vi "Filter Data.vi"(7 "k (0.7)":dbl=0.7 format="%#_13g", 10 "High Filter k (0.5)":dbl=0.5 format="%#_13g", 11 "Raw Acq Data in in":T1) -> (3 "Raw Acq Data out":T1)   [LabVIEW 2018, in "RT - Analysis.lvlib"]
doc: "Filters the following data sets:\n00-00, 00-01, 00-03\n01-00, 01-01, 01-02\n02-02, 02-03, 02-05"
uses:
  RT - Analysis.lvlib
  Top Level/Shared Controls/Acq Data.ctl
  Public VIs/First Order Lag Filter (1D DBL).vi
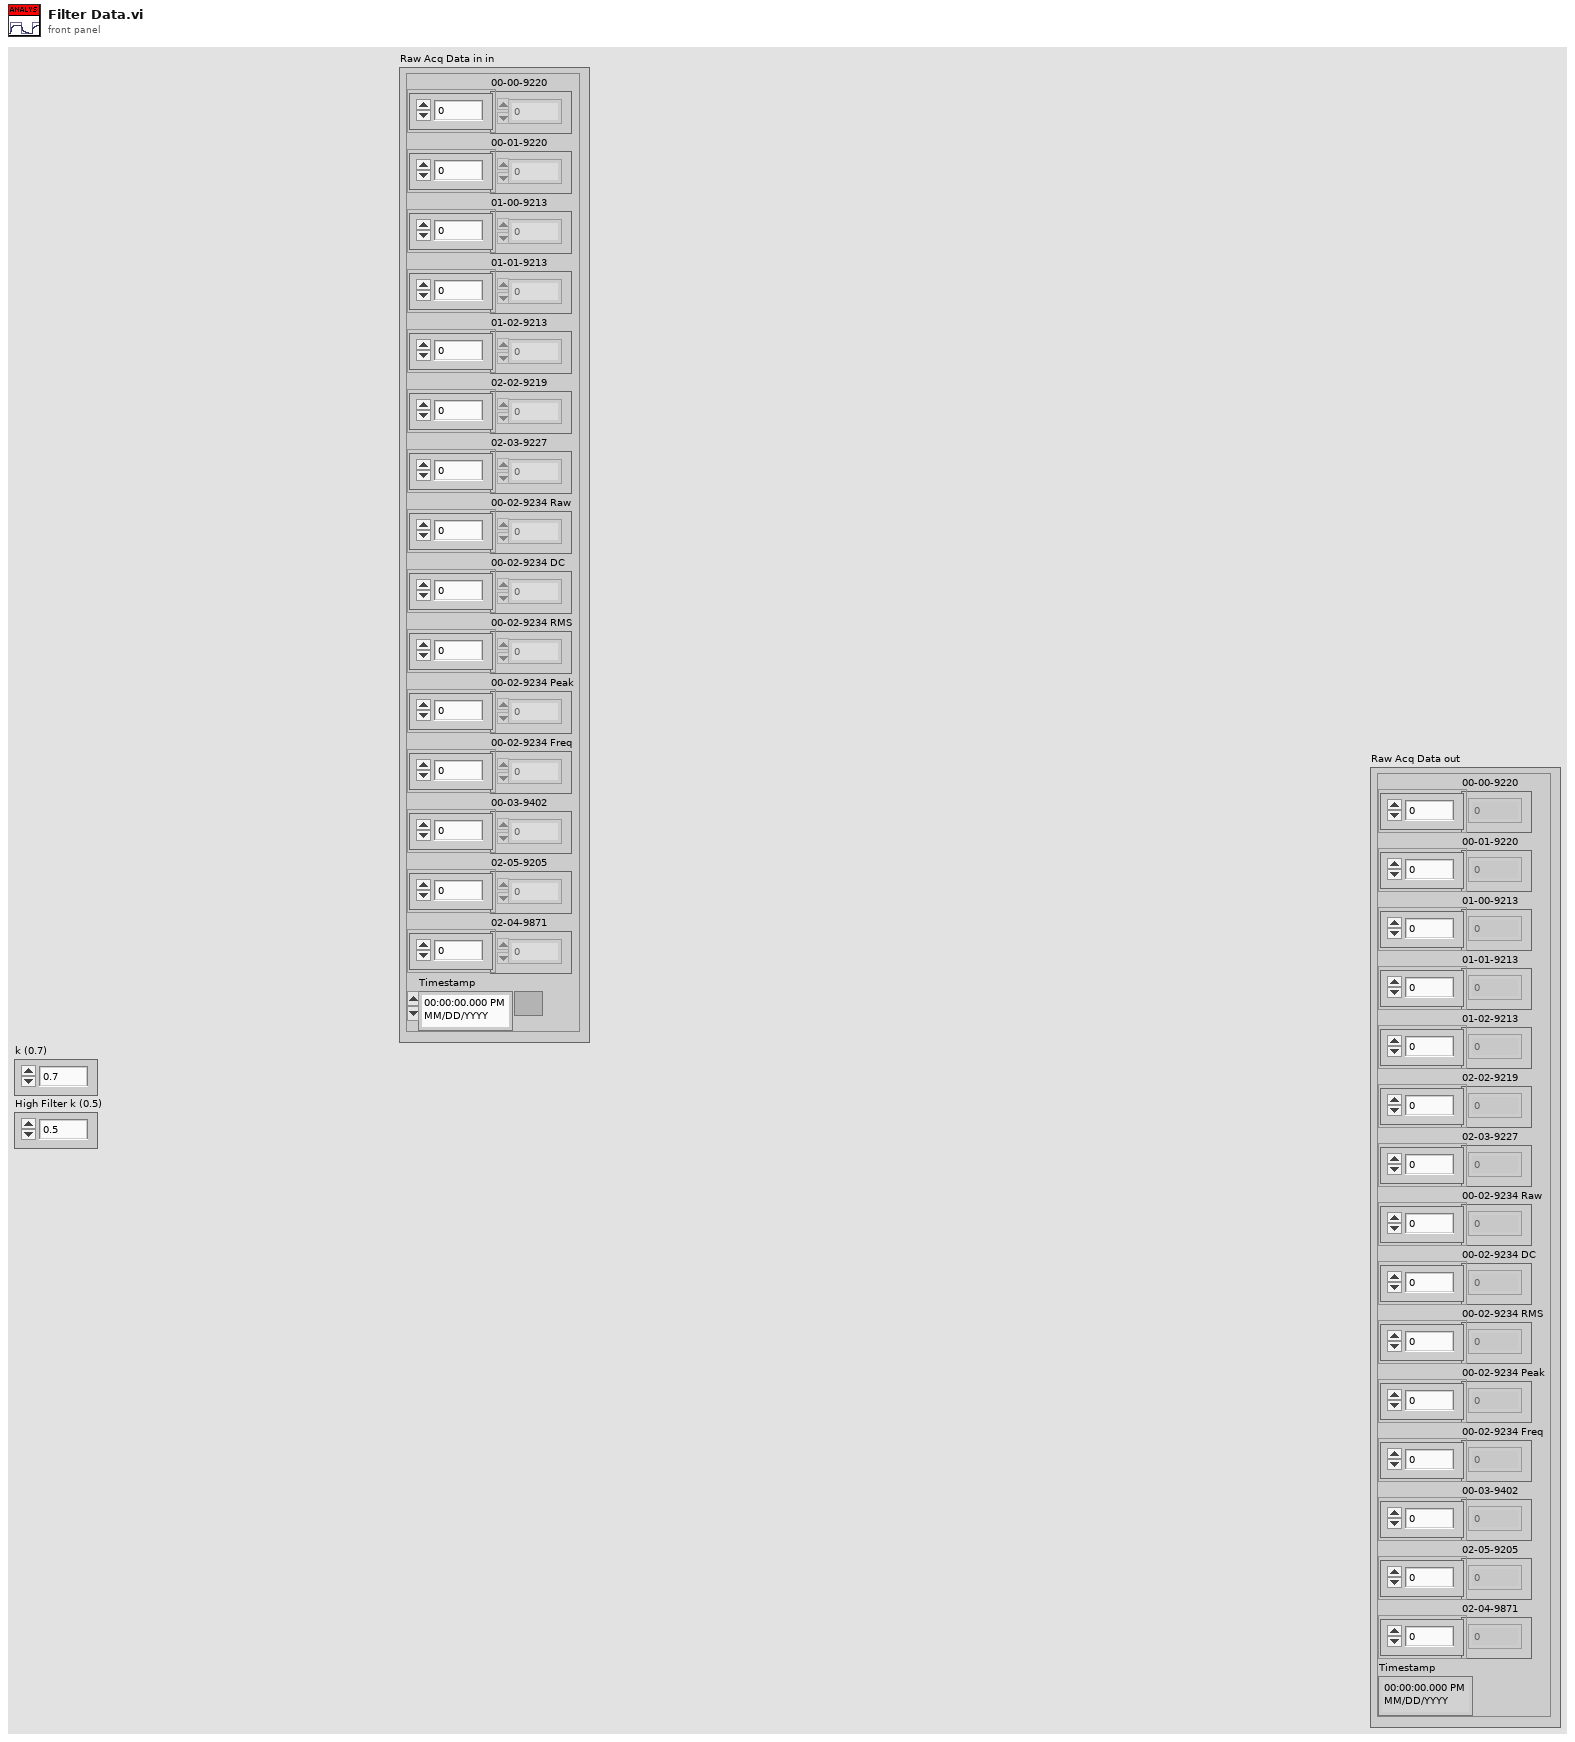
[diagram p1: front panel]
types:
  T1 = typedef "Acq Data.ctl" = cluster{"00-00-9220":dbl[], "00-01-9220":dbl[], "01-00-9213":dbl[], "01-01-9213":dbl[], "01-02-9213":dbl[], "02-02-9219":dbl[], "02-03-9227":dbl[], "00-02-9234 Raw":dbl[], "00-02-9234 DC":dbl[], "00-02-9234 RMS":dbl[], "00-02-9234 Peak":dbl[], "00-02-9234 Freq":dbl[], "00-03-9402":dbl[], "02-05-9205":dbl[], "02-04-9871":dbl[], "Timestamp":timestamp}
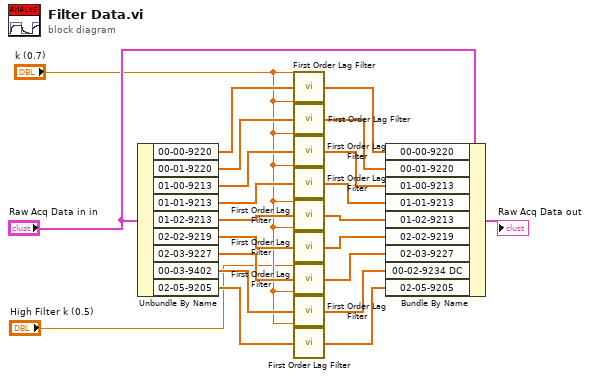
[diagram p0: block diagram]
diagram:
  n1 = Unbundle By Name("Raw Acq Data in in") -> ("00-00-9220"=w20:dbl[], "00-01-9220"=w19:dbl[], "01-00-9213"=w12:dbl[], "01-01-9213"=w18:dbl[], "01-02-9213"=w13:dbl[], "02-02-9219"=w17:dbl[], "02-03-9227"=w16:dbl[], "00-03-9402"=w15:dbl[], "02-05-9205"=w14:dbl[])
  n2 = call-poly "First Order Lag Filter.vi"("k (1)"="k (0.7)", "Raw Values in"=w20) -> ("Filtered Values out"=w10:dbl[])  [unwired: 5 in]
  n3 = call-poly "First Order Lag Filter.vi"("k (1)"="k (0.7)", "Raw Values in"=w19) -> ("Filtered Values out"=w9:dbl[])  [unwired: 5 in]
  n4 = call-poly "First Order Lag Filter.vi"("k (1)"="k (0.7)", "Raw Values in"=w12, "Prev Filtered Vals (Optional)"=w12) -> ("Filtered Values out"=w8:dbl[])  [unwired: 4 in]
  n5 = call-poly "First Order Lag Filter.vi"("k (1)"="k (0.7)", "Raw Values in"=w18) -> ("Filtered Values out"=w7:dbl[])  [unwired: 5 in]
  n6 = call-poly "First Order Lag Filter.vi"("k (1)"="k (0.7)", "Raw Values in"=w13) -> ("Filtered Values out"=w2:dbl[])  [unwired: 5 in]
  n7 = call-poly "First Order Lag Filter.vi"("k (1)"="k (0.7)", "Raw Values in"=w17) -> ("Filtered Values out"=w6:dbl[])  [unwired: 5 in]
  n8 = call-poly "First Order Lag Filter.vi"("k (1)"="High Filter k (0.5)", "Raw Values in"=w16) -> ("Filtered Values out"=w5:dbl[])  [unwired: 5 in]
  n9 = call-poly "First Order Lag Filter.vi"("k (1)"="k (0.7)", "Raw Values in"=w15) -> ("Filtered Values out"=w4:dbl[])  [unwired: 5 in]
  n10 = call-poly "First Order Lag Filter.vi"("k (1)"="k (0.7)", "Raw Values in"=w14) -> ("Filtered Values out"=w3:dbl[])  [unwired: 5 in]
  n11 = Bundle By Name(cluster="Raw Acq Data in in", "00-00-9220"=w10, "00-01-9220"=w9, "01-00-9213"=w8, "01-01-9213"=w7, "01-02-9213"=w2, "02-02-9219"=w6, "02-03-9227"=w5, "00-02-9234 DC"=w4, "02-05-9205"=w3) -> (→"Raw Acq Data out":T1)
